vi "Center Dialog on Caller.vi"(8 "error in (no error)":errorcluster, 9 "Dialog VI":refnum<vi>, 11 "Calling VI in":refnum<vi>) -> (0 "error out":errorcluster, 1 "Dialog VI out":refnum<vi>)   [LabVIEW 2020, in "VI Properties Editor.lvlib"]
doc: "Centers the front panel of a dialog VI in relation to the calling VI."
uses:
  VI Properties Editor.lvlib
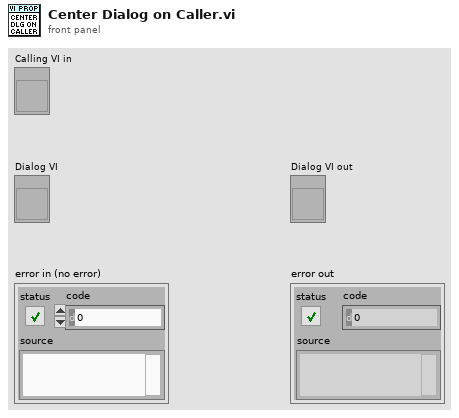
[diagram p1: front panel]
types:
  T1 = typedef "LVAllMonitorsDisplayTypeDef.ctl" = cluster{"Bounds":cluster{"Left":i16, "Top":i16, "Right":i16, "Bottom":i16}, "Depth":i16}[]
  T2 = typedef "LVRectTypeDef.ctl" = cluster{"Left":i16, "Top":i16, "Right":i16, "Bottom":i16}
  T3 = cluster{"left":i16, "top":i16, "right":i16, "bottom":i16}
  T4 = cluster{"Bounds":cluster{"Left":i16, "Top":i16, "Right":i16, "Bottom":i16}, "Depth":i16}
  T5 = cluster{"Left":i16, "Top":i16, "Right":i16, "Bottom":i16}
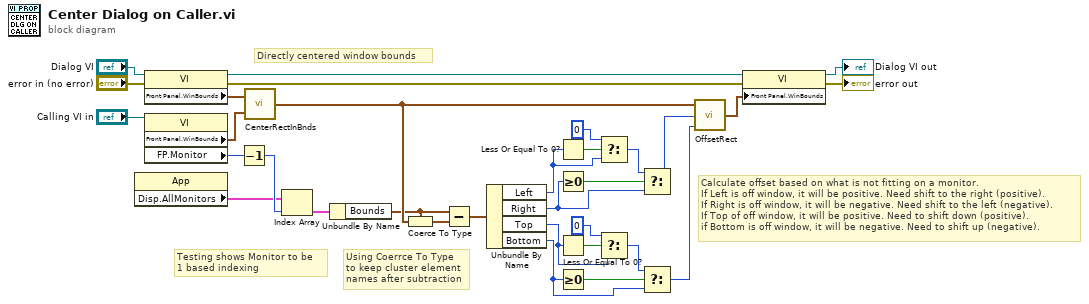
[diagram p0: block diagram]
diagram:
  # "Testing shows Monitor to be\n1 based indexing"
  # "Directly centered window bounds"
  # "Calculate offset based on what is not fitting on a monitor.\nIf Left is off window, it will be positive. Need shift to the right (positive).\nIf Right is off window, it will be negative. Need shift to the left (negative).\nIf Top of off window, it will be positive. Need to shift down (positive).\nif Bottom is off window, it will be negative. Need to shift up (negative)."
  # "Using Coerrce To Type\nto keep cluster element\nnames after subtraction"
  n1 = property class="App"() -> ("Disp.AllMonitors"=w12:T1)  [unwired: 2 in, 2 out]
  n2 = property class="VI"(reference="Dialog VI", error in="error in (no error)") -> (reference out=w7:refnum<vi>, error out=w32:errorcluster, "Front Panel.WinBounds"=w9:T2)
  n3 = property class="VI"(reference="Calling VI in") -> ("Front Panel.WinBounds"=w5:T2, "FP.Monitor"=w10:u16)  [unwired: 1 in, 2 out]
  n4 = Decrement(x=w10) -> (x-1=w13:u16)
  n5 = call <vilib>:"CenterRectInBnds.vi"("bounds"=w5, "rect"=w9) -> ("centered rect"=w31:T3)
  n6 = Index Array(array=w12, index=w13) -> (element=w11:T4)
  n7 = Unbundle By Name(w11) -> ("Bounds"=w15:T5)
  n8 = Coerce To Type(0:w31, 1:w15) -> (2:w14:T5)
  n9 = Subtract(x=w15, y=w14) -> (x-y=w16:T5)
  n10 = Unbundle By Name(w16) -> ("Left"=w4:i16, "Right"=w21:i16, "Top"=w26:i16, "Bottom"=w27:i16)
  n11 = Less Or Equal To 0?(x=w4) -> (x <= 0?=w17:bool)
  n12 = Greater Or Equal To 0?(x=w21) -> (x >= 0?=w19:bool)
  n13 = Less Or Equal To 0?(x=w26) -> (x <= 0?=w25:bool)
  n14 = Greater Or Equal To 0?(x=w27) -> (x >= 0?=w23:bool)
  n15 = Select(t=i16 0 ("Left"), s=w17, f=w4) -> (s? t:f=w20:i16)
  n16 = Select(t=i16 0 ("Left"), s=w25, f=w26) -> (s? t:f=w22:i16)
  n17 = Select(t=w20, s=w19, f=w21) -> (s? t:f=w29:i16)
  n18 = Select(t=w22, s=w23, f=w27) -> (s? t:f=w30:i16)
  n19 = call <vilib>:"OffsetRect.vi"("v"=w30, "h"=w29, "rect"=w31) -> ("offset rect"=w28:T3)
  n20 = property class="VI"(reference=w7, error in=w32, "Front Panel.WinBounds"=w28) -> (reference out=→"Dialog VI out":refnum<vi>, error out=→"error out":errorcluster)
